vi "Buffer Scans.vi"(6 "Local Data":T1, 8 "error in":errorcluster, 11 "Acquisition Scan":T2) -> (0 "error out":errorcluster, 4 "Local Data Out":T1)   [LabVIEW 2025]
uses:
  Controls/Acquisition Packet.ctl
  Controls/Local Data_Display.ctl
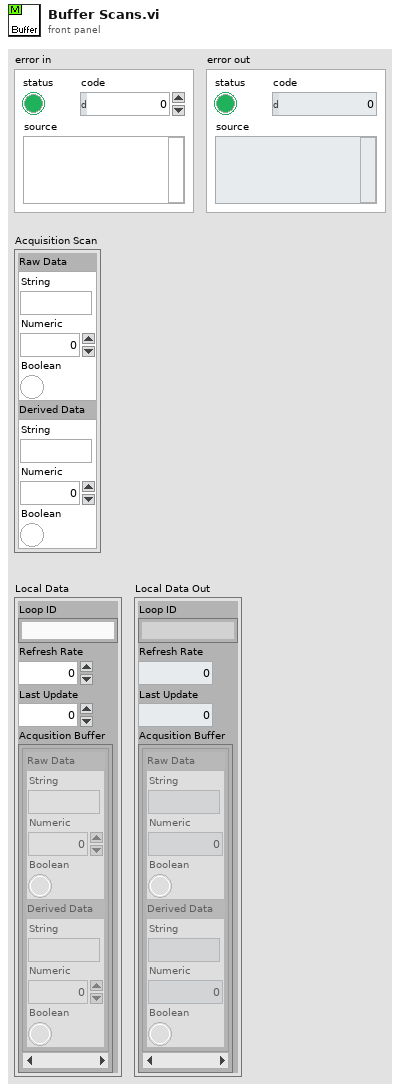
[diagram p1: front panel]
types:
  T1 = typedef "Local Data_Display.ctl" = cluster{"Loop ID":string, "Refresh Rate":dbl, "Last Update":dbl, "Acqusition Buffer":T2[]}
  T2 = typedef "Acquisition Packet.ctl" = cluster{"Raw Data":cluster{"String":string, "Numeric":dbl, "Boolean":bool}, "Derived Data":cluster{"String":string, "Numeric":dbl, "Boolean":bool}}
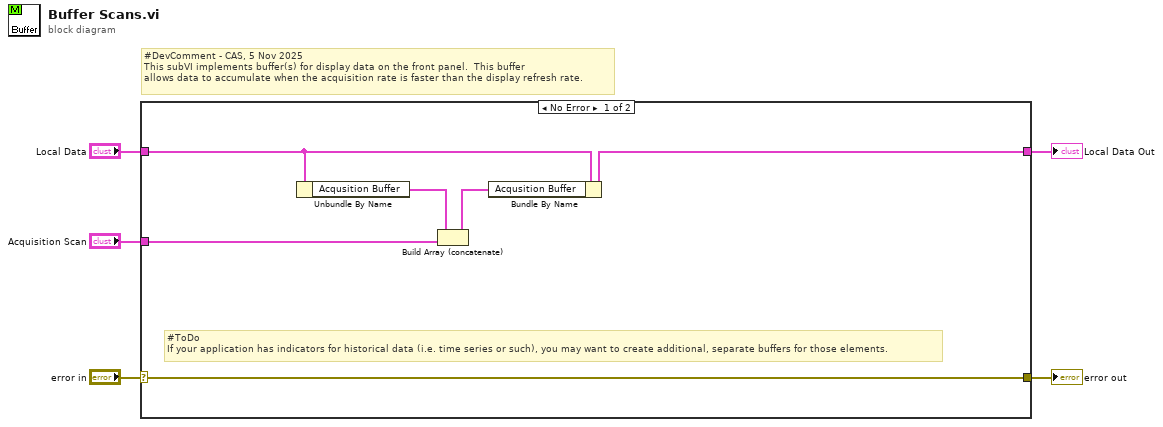
[diagram p0: block diagram]
diagram:
  # "#DevComment - CAS, 5 Nov 2025\nThis subVI implements buffer(s) for display data on the front panel.  This buffer\nallows data to accumulate when the acquisition rate is faster than the display refresh rate."
  n1 = case shown="No Error" "error in" {
    selector: "error in" -> [w6 w12]
    tunnel: "Acquisition Scan" -> [w8 _]
    tunnel: "Local Data" -> [w11 w13]
    tunnel: [w7 w13] -> w2
    tunnel: [w6 w12] -> w1
    frame No Error {
      # "#ToDo\nIf your application has indicators for historical data (i.e. time series or such), you may want to create additional, separate buffers for those elements."
      n2 = Unbundle By Name(w11) -> ("Acqusition Buffer"=w10:T2[])
      n3 = Build Array (concatenate)(w10, w8) -> (w9:T2[])
      n4 = Bundle By Name(cluster=w11, "Acqusition Buffer"=w9) -> (w7:T1)
    }
    frame Error {
    }
  }
  "error out" <- w1
  "Local Data Out" <- w2
